vi "Generate Simulated Data.vi"(7 "Error In":errorcluster, 10 "Signal Type":T1) -> (0 "Error Out":errorcluster, 2 "Graph Data":waveform(dbl)[](array[waveform]))   [LabVIEW 2020]
doc: "Generates sample waveforms according to the signal type in the HW Config input."
uses:
  Typedefs/Signal Type.ctl
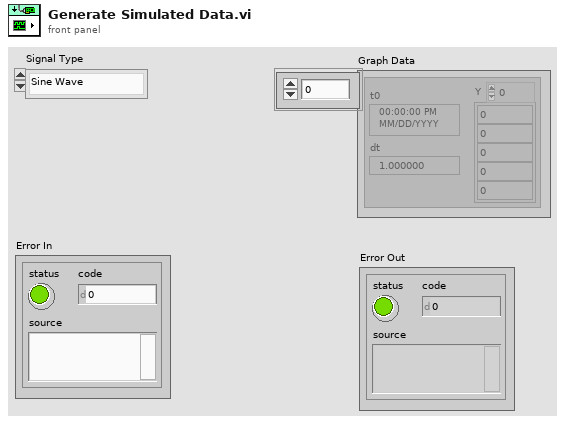
[diagram p1: front panel]
types:
  T1 = typedef "Signal Type.ctl" = enum16{"Sine Wave", "Square with Noise"}
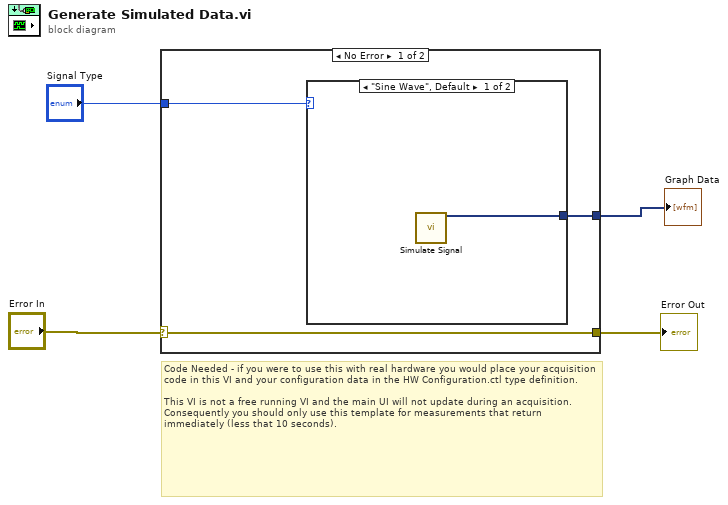
[diagram p0: block diagram]
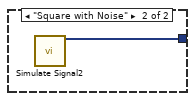
[diagram p2: hidden frame]
diagram:
  # "Code Needed - if you were to use this with real hardware you would place your acquisition code in this VI and your configuration data in the HW Configuration.ctl type definition.\n\nThis VI is not a free running VI and the main UI will not update during an acquisition.  Consequently you should only use this template for measurements that return immediately (less that 10 seconds)."
  n1 = case shown="No Error" "Error In" {
    selector: "Error In" -> [w7 w10]
    tunnel: [w7 w10] -> w3
    tunnel: [w6 _] -> w1
    tunnel: "Signal Type" -> [w5 _]
    frame No Error {
      n2 = case shown="\"Sine Wave\", Default" w5 {
        tunnel: [w8 w9] -> w6
        frame "Sine Wave", Default {
          n3 = call "Simulate Signal"() -> ("Sine"=w8:dynamicdata)  [unwired: 14 in, 1 out]
        }
        frame "Square with Noise" {
          n4 = call "Simulate Signal2"() -> ("Square with Noise"=w9:dynamicdata)  [unwired: 14 in, 1 out]
        }
      }
    }
    frame Error {
    }
  }
  "Error Out" <- w3
  "Graph Data" <- w1
